vi "Initialize Aliases Page.vi"(8 "error in (no error)":errorcluster, 10 "Aliases Page Controls":T1, 11 "Aliases Ref in":T2 format="%.0x") -> (0 "error out":errorcluster, 3 "Aliases Ref out":T2 format="%.0x")   [LabVIEW 2020, in "Routing and Faulting System Explorer.lvlib"]
uses:
  Routing and Faulting System Explorer.lvlib
  <vilib>/NI VeriStand/Custom Device API/Custom Device Item Ref.ctl
  Aliases Page Controls.ctl
  Alias.ctl
  Endpoint.ctl
  Form Endpoint.vi
  Scripting/Routing and Faulting Scripting.lvlib
  <vilib>/NI VeriStand/Custom Device API/Custom Device API.lvlib
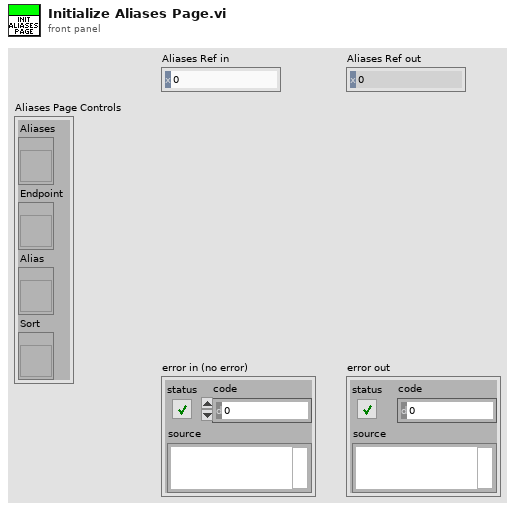
[diagram p1: front panel]
types:
  T1 = typedef "Routing and Faulting System Explorer.lvlib/Aliases Page Controls.ctl" = cluster{"Aliases":refnum<vi>, "Endpoint":refnum<vi>, "Alias":refnum<vi>, "Sort":refnum<vi>}
  T2 = typedef "Custom Device API.lvlib/Custom Device Item Ref.ctl" = u64
  T3 = enum8{"Enabled", "Disabled", "Disabled and Grayed Out"}
  T4 = typedef "Routing and Faulting Shared.lvlib/Alias Mapping.ctl" = cluster{"Alias":string, "Endpoint":T5}
  T5 = typedef "Routing and Faulting Shared.lvlib/Alias Endpoint.ctl" = cluster{"Module Path":string, "Endpoint":string}
  T6 = typedef "Routing and Faulting System Explorer.lvlib/Alias.ctl" = cluster{"Endpoint":T7, "Alias":string, "Remove":bool}
  T7 = typedef "Routing and Faulting System Explorer.lvlib/Endpoint.ctl" = string
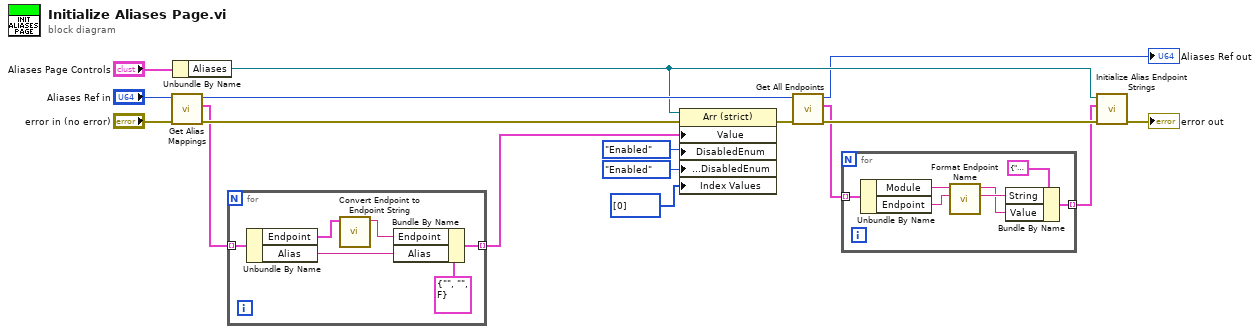
[diagram p0: block diagram]
diagram:
  n1 = call "Get Alias Mappings.vi"("error in"="error in (no error)", "endpoint aliases in"="Aliases Ref in") -> ("error out"=w12:errorcluster, "alias mappings"=w11:T4[], "endpoint aliases out"=w8:T2)  [unwired: 7 in]
  n2 = Unbundle By Name("Aliases Page Controls") -> ("Aliases"=w5:refnum<vi>)
  n3 = for {
    tunnel: w11 -> [w21] mode=indexing
    tunnel: [w20] -> w9 mode=indexing
    n4 = Unbundle By Name(w21) -> ("Endpoint"=w19:T5, "Alias"=w23:string)
    n5 = call "Convert Endpoint to Endpoint String.vi"("Endpoint"=w19) -> ("Endpoint String"=w18:string)  [unwired: 10 in]
    n6 = Bundle By Name(cluster=T6 {"Endpoint"="", "Alias"="", "Remove"=FALSE} ("Alias"), "Endpoint"=w18, "Alias"=w23) -> (w20:T6)
  }
  n7 = property class="Arr (strict)"(reference=w5, error in=w12, "Value"=w9, "DisabledEnum"=T3."Enabled" ("Disabled"), "Array Element.DisabledEnum"=T3."Enabled" ("Array Element.Disabled"), "Index Values"=u32[] [0]) -> (error out=w7:errorcluster)  [unwired: 1 out]
  n8 = call "Get All Endpoints.vi"("error in (no error)"=w7, "Aliases Ref in"=w8) -> ("error out"=w6:errorcluster, "Addressable Endpoints"=w2:cluster{"Module":string, "Endpoint":string}[], "Aliases Ref out"=→"Aliases Ref out":T2)  [unwired: 7 in]
  n9 = for {
    tunnel: w2 -> [w30] mode=indexing
    tunnel: [w25] -> w1 mode=indexing
    n10 = Unbundle By Name(w30) -> ("Module"=w29:string, "Endpoint"=w28:string)
    n11 = call "Format Endpoint Name.vi"("Endpoint"=w28, "Module Path"=w29) -> ("Formatted Endpoint Name"=w27:string, "Full Endpoint Name"=w26:string)  [unwired: 8 in]
    n12 = Bundle By Name(cluster=cluster{"String":string, "Value":string} {"String"="", "Value"=""}, "String"=w27, "Value"=w26) -> (w25:cluster{"String":string, "Value":string})
  }
  n13 = call "Initialize Alias Endpoint Strings.vi"("error in (no error)"=w6, "Endpoints"=w1, "Aliases Ctl Ref"=w5) -> ("error out"=→"error out":errorcluster)  [unwired: 7 in, 1 out]
